vi "motor-Open-v2.vi"(8 "Error In":errorcluster, 10 "S/N Motor":string(combo), 11 "ref Boolean in":refnum<vi>) -> (0 "Error Out":errorcluster, 2 "Motor Status":bool=TRUE, 3 "Refnum out":refnum<k7>)   [LabVIEW 2014]
doc: "This VI open Thorlab Motors and check if everything is Ok \n\nAndré Romero - 2023\nandretec@ifsc.usp.br\nIFSC - USP"
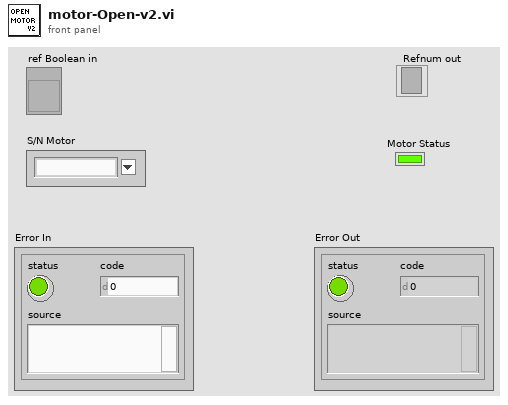
[diagram p1: front panel]
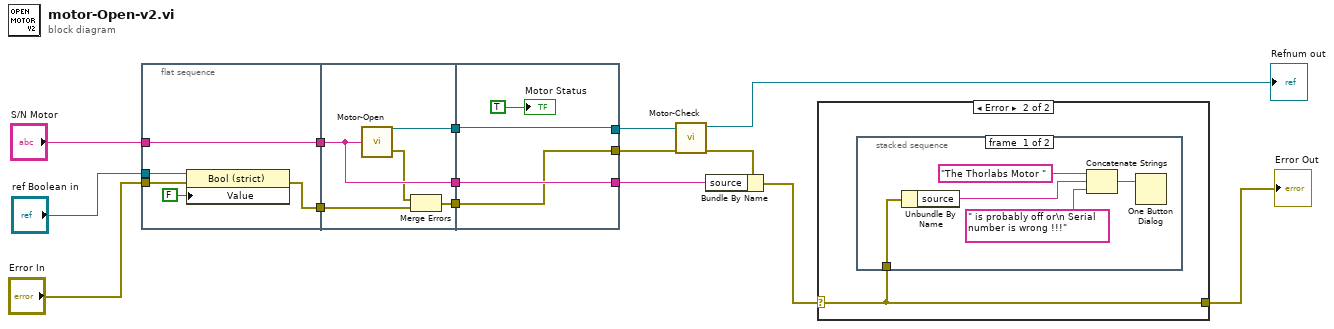
[diagram p0: block diagram]
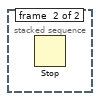
[diagram p3: hidden frame]
diagram:
  n1 = flat-sequence {
    tunnel: "ref Boolean in" -> [w19]
    tunnel: "S/N Motor" -> [w20]
    tunnel: [w20] -> w13
    tunnel: "Error In" -> [w17]
    tunnel: [w16] -> w2
    tunnel: [w25] -> w14
    tunnel: w13 -> [w24]
    tunnel: [w24] -> w9
    tunnel: w2 -> [w22]
    tunnel: [w21] -> w1
    tunnel: [w29] -> w10
    tunnel: [w26] -> w11
    tunnel: w14 -> [w29]
    tunnel: [w27] -> w7
    tunnel: w9 -> [w27]
    tunnel: w1 -> [w26]
    frame #0 {
      n2 = property class="Bool (strict)"(reference=w19, error in=w17, "Value"=FALSE) -> (error out=w16:errorcluster)  [unwired: 1 out]
    }
    frame #1 {
      n3 = call "Motor-Open.vi"("S/N Motor"=w24) -> ("MG17Motor 2"=w25:refnum<k7>, "error out"=w23:errorcluster)
      n4 = Merge Errors(w23, w22) -> (w21:errorcluster)
    }
    frame #2 {
      "Motor Status" <- TRUE ("Motor3\nLigado")
    }
  }
  n5 = call "Motor-Check.vi"("error in (no error)"=w11, "Automation Refnum in"=w10) -> ("error out"=w8:errorcluster, "Automation Refnum out"=→"Refnum out":refnum<k7>)  [unwired: 8 in]
  n6 = Bundle By Name(cluster=w8, "source"=w7) -> (w5:errorcluster)
  n7 = case shown="Error" w5 {
    selector: w5 -> [w30 w31]
    tunnel: [w30 w31] -> w4
    frame No Error {
    }
    frame Error {
      n8 = stacked-sequence {
        tunnel: w31 -> [w36 _]
        frame #0 {
          n9 = Unbundle By Name(w36) -> ("source"=w34:string)
          n10 = Concatenate Strings("The Thorlabs Motor " ("message"), w34, " is probably off or\n Serial number is wrong !!!") -> (w33:string)
          n11 = One Button Dialog(message=w33) -> ()  [unwired: 1 in, 1 out]
        }
        frame #1 {
          n12 = Stop() -> ()  [unwired: 1 in]
        }
      }
    }
  }
  "Error Out" <- w4
